vi "descriptors.vi"(10 "# of channels":i32=4) -> (1 "# of channels":i32, 3 "channel #s":i32[](array[numeric]), 5 "mount pairs":cluster{i32, i32}[](array[cluster]), 7 "DAQ channels":string[](array[string]))   [LabVIEW 2020]
panel:
  out "mount pairs XY":cluster{"X":i32, "Y":i32}[](array[cluster])
  out "device channels":string[](array[string])
  out "mounts":string[](array[string])
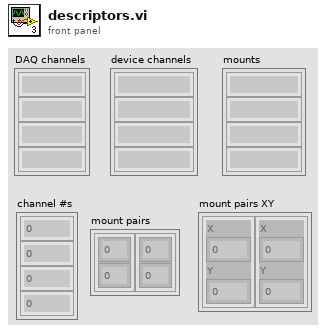
[diagram p1: front panel]
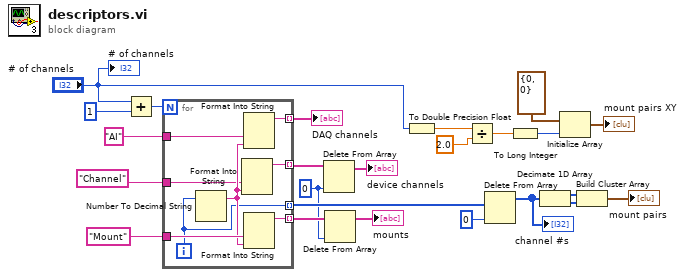
[diagram p0: block diagram]
diagram:
  w3 = 0 ("index")
  n1 = Add(x="# of channels", y=1) -> (x+y=w20:i32)
  n2 = for {
    N: w20 -> [_]
    tunnel: [w25] -> w18 mode=indexing
    tunnel: "Mount" -> [w32]
    tunnel: [w31] -> w14 mode=indexing
    tunnel: "AI" -> [w28]
    tunnel: [w27] -> w16 mode=indexing
    tunnel: "Channel" -> [w29]
    tunnel: [w26] -> w7 mode=indexing
    i -> [w25]
    n3 = Number To Decimal String(number=w25) -> (decimal integer string=w30:string)  [unwired: 1 in]
    n4 = Format Into String(w29, w30) -> (resulting string=w26:string)  [unwired: 3 in, 1 out]
    n5 = Format Into String(w28, w30) -> (resulting string=w27:string)  [unwired: 3 in, 1 out]
    n6 = Format Into String(w32, w30) -> (resulting string=w31:string)  [unwired: 3 in, 1 out]
  }
  "DAQ channels" <- w16
  n7 = Delete From Array(array=w7, index=w3) -> (array with subset deleted=→"device channels":string[])  [unwired: 1 in, 1 out]
  n8 = Delete From Array(array=w14, index=w3) -> (array with subset deleted=→"mounts":string[])  [unwired: 1 in, 1 out]
  n9 = To Double Precision Float(number="# of channels") -> (double precision float=w2:dbl)
  n10 = Divide(x=w2, y=2.0) -> (x/y=w5:dbl)
  n11 = Delete From Array(array=w18, index=0) -> (array with subset deleted=w24:i32[])  [unwired: 1 in, 1 out]
  "channel #s" <- w24
  n12 = To Long Integer(number=w5) -> (32bit integer=w10:i32)
  n13 = Decimate 1D Array(w24) -> (w21:i32[], w22:i32[])
  n14 = Initialize Array ("Mounts")(cluster{"X":i32, "Y":i32} {"X"=0, "Y"=0}, w10) -> (→"mount pairs XY":cluster{"X":i32, "Y":i32}[])
  n15 = Build Cluster Array(w21, w22) -> (→"mount pairs":cluster{i32, i32}[])
  "# of channels" <- "# of channels"
